vi "Quadrotor RT.vi"() -> ()   [LabVIEW 2015]
uses:
  <vilib>/Platform/TimedLoop/XDataNode/timing_clust.ctl
  <vilib>/Platform/TimedLoop/XDataNode/nitl_modes.ctl
  <vilib>/Platform/TimedLoop/XDataNode/wakeup.ctl
  <vilib>/FPGAPlugInAG/myRIO-1900/niLvFpga_Open_myRIO-1900.vi
  <vilib>/rvi/interface/common/dynamic/niFpgaDynamicAddResources.vi
  <vilib>/myRIO/Common/Instrument Driver Framework/Utilities/vis/FPGA Ref Manager.vi
  <vilib>/Utility/error.llb/Error Cluster From Error Code.vi
  <vilib>/myRIO/Common/Instrument Driver Framework/Utilities/vis/Ref Counter.vi
  <vilib>/Utility/xml.llb/Read From XML File(string).vi
  <vilib>/Utility/xml.llb/Write to XML File(string).vi
  <vilib>/FPGAPlugInAG/Dynamic/niLvFpga_Close_Dynamic.vi
  <vilib>/rvi/interface/nirviOpenFPGA/nirviOpenFPGA.xnode
  FPGA Bitfiles/MyThirdNImyRIOPr_FPGATarget_myRIO-1900Quadro_oM0Jv1TSYjE.lvbitx
  <vilib>/Platform/TimedLoop/XDataNode/XDataNode.xnode
  <vilib>/rvi/interface/nirviCloseFPGA/nirviCloseFPGA.xnode
  <vilib>/Platform/TimedLoop/XDataNode/XDNodeRunTimeDep.lvlib
  <vilib>/myRIO/Instrument Drivers/Utilities/Utilities.lvlib
panel:
  out "Buffer In":u8[](array[numeric])=[204, 0, 0, 0, 0, 0, 0, 0, 0, 0, 0, 0, 0, 0, 0, 0, 0, 0, 0, 0, 0, 0, 0, 0, 0, 0, 0, 0, 0, 0, 0, 0, 85, 170] format="0x%x"
  in  "停止调试":bool
  out "roll":dbl(knob) scale=-90.0..90.0
  out "陀螺仪积分时间间隔":sgl(graph)=0.002
  in  "D":dbl(slide)=45.4945 scale=0.0..300.0
  in  "P":dbl(slide)=50.5495 scale=0.0..500.0
  in  "I":dbl(slide)=0.013 scale=0.0..5.0
  in  "Yaw_D":dbl=10.0
  in  "Yaw_I":dbl
  in  "Yaw_P":dbl=200.0
  in  "滑动杆":dbl(slide)=-0.061919504643962814 scale=-10.0..10.0
  out "Pitch: 控制\\反馈":cluster{sgl, "Pitch":dbl}(graph)
  out "Roll: 控制\\反馈":cluster{sgl, "Roll":dbl}(graph)
  out "Yaw: 控制\\反馈":cluster{"GYR_I_Z":sgl}(graph)
  out "Roll计算后数值":dbl
  out "Pitch计算后数值":dbl
  out "Yaw计算后数值":dbl
  out "输出簇":T1(graph)
  in  "ACCADJ":T2
  out "GYR_I_X":sgl
  out "GYR_I_Y":sgl
  out "AccMean":T2={"ACC_OFFSET_X"=63.977, "ACC_OFFSET_Y"=220.058, "ACC_OFFSET_Z"=0.0}
  out "GyrMean":T3
  out "摇杆按键 9":bool[](array[boolean])
  out "摇杆按键 8":bool[](array[boolean])
  out "摇杆按键 7":bool[](array[boolean])
  out "摇杆按键 6":bool[](array[boolean])
  out "摇杆按键 5":bool[](array[boolean])
  out "摇杆按键 4":bool[](array[boolean])
  out "摇杆按键 3":bool[](array[boolean])
  out "摇杆按键 2":bool[](array[boolean])
  out "油门":u16(knob) scale=0.0..20000.0
  out "X axis":i32(slide) scale=-32768.0..32767.0
  out "Y axis":i32(slide) scale=-32768.0..32767.0
  out "小方向":u8
  out "摇杆按键":bool[](array[boolean])
  out "XY图":cluster{i32[], i32[]}(graph)
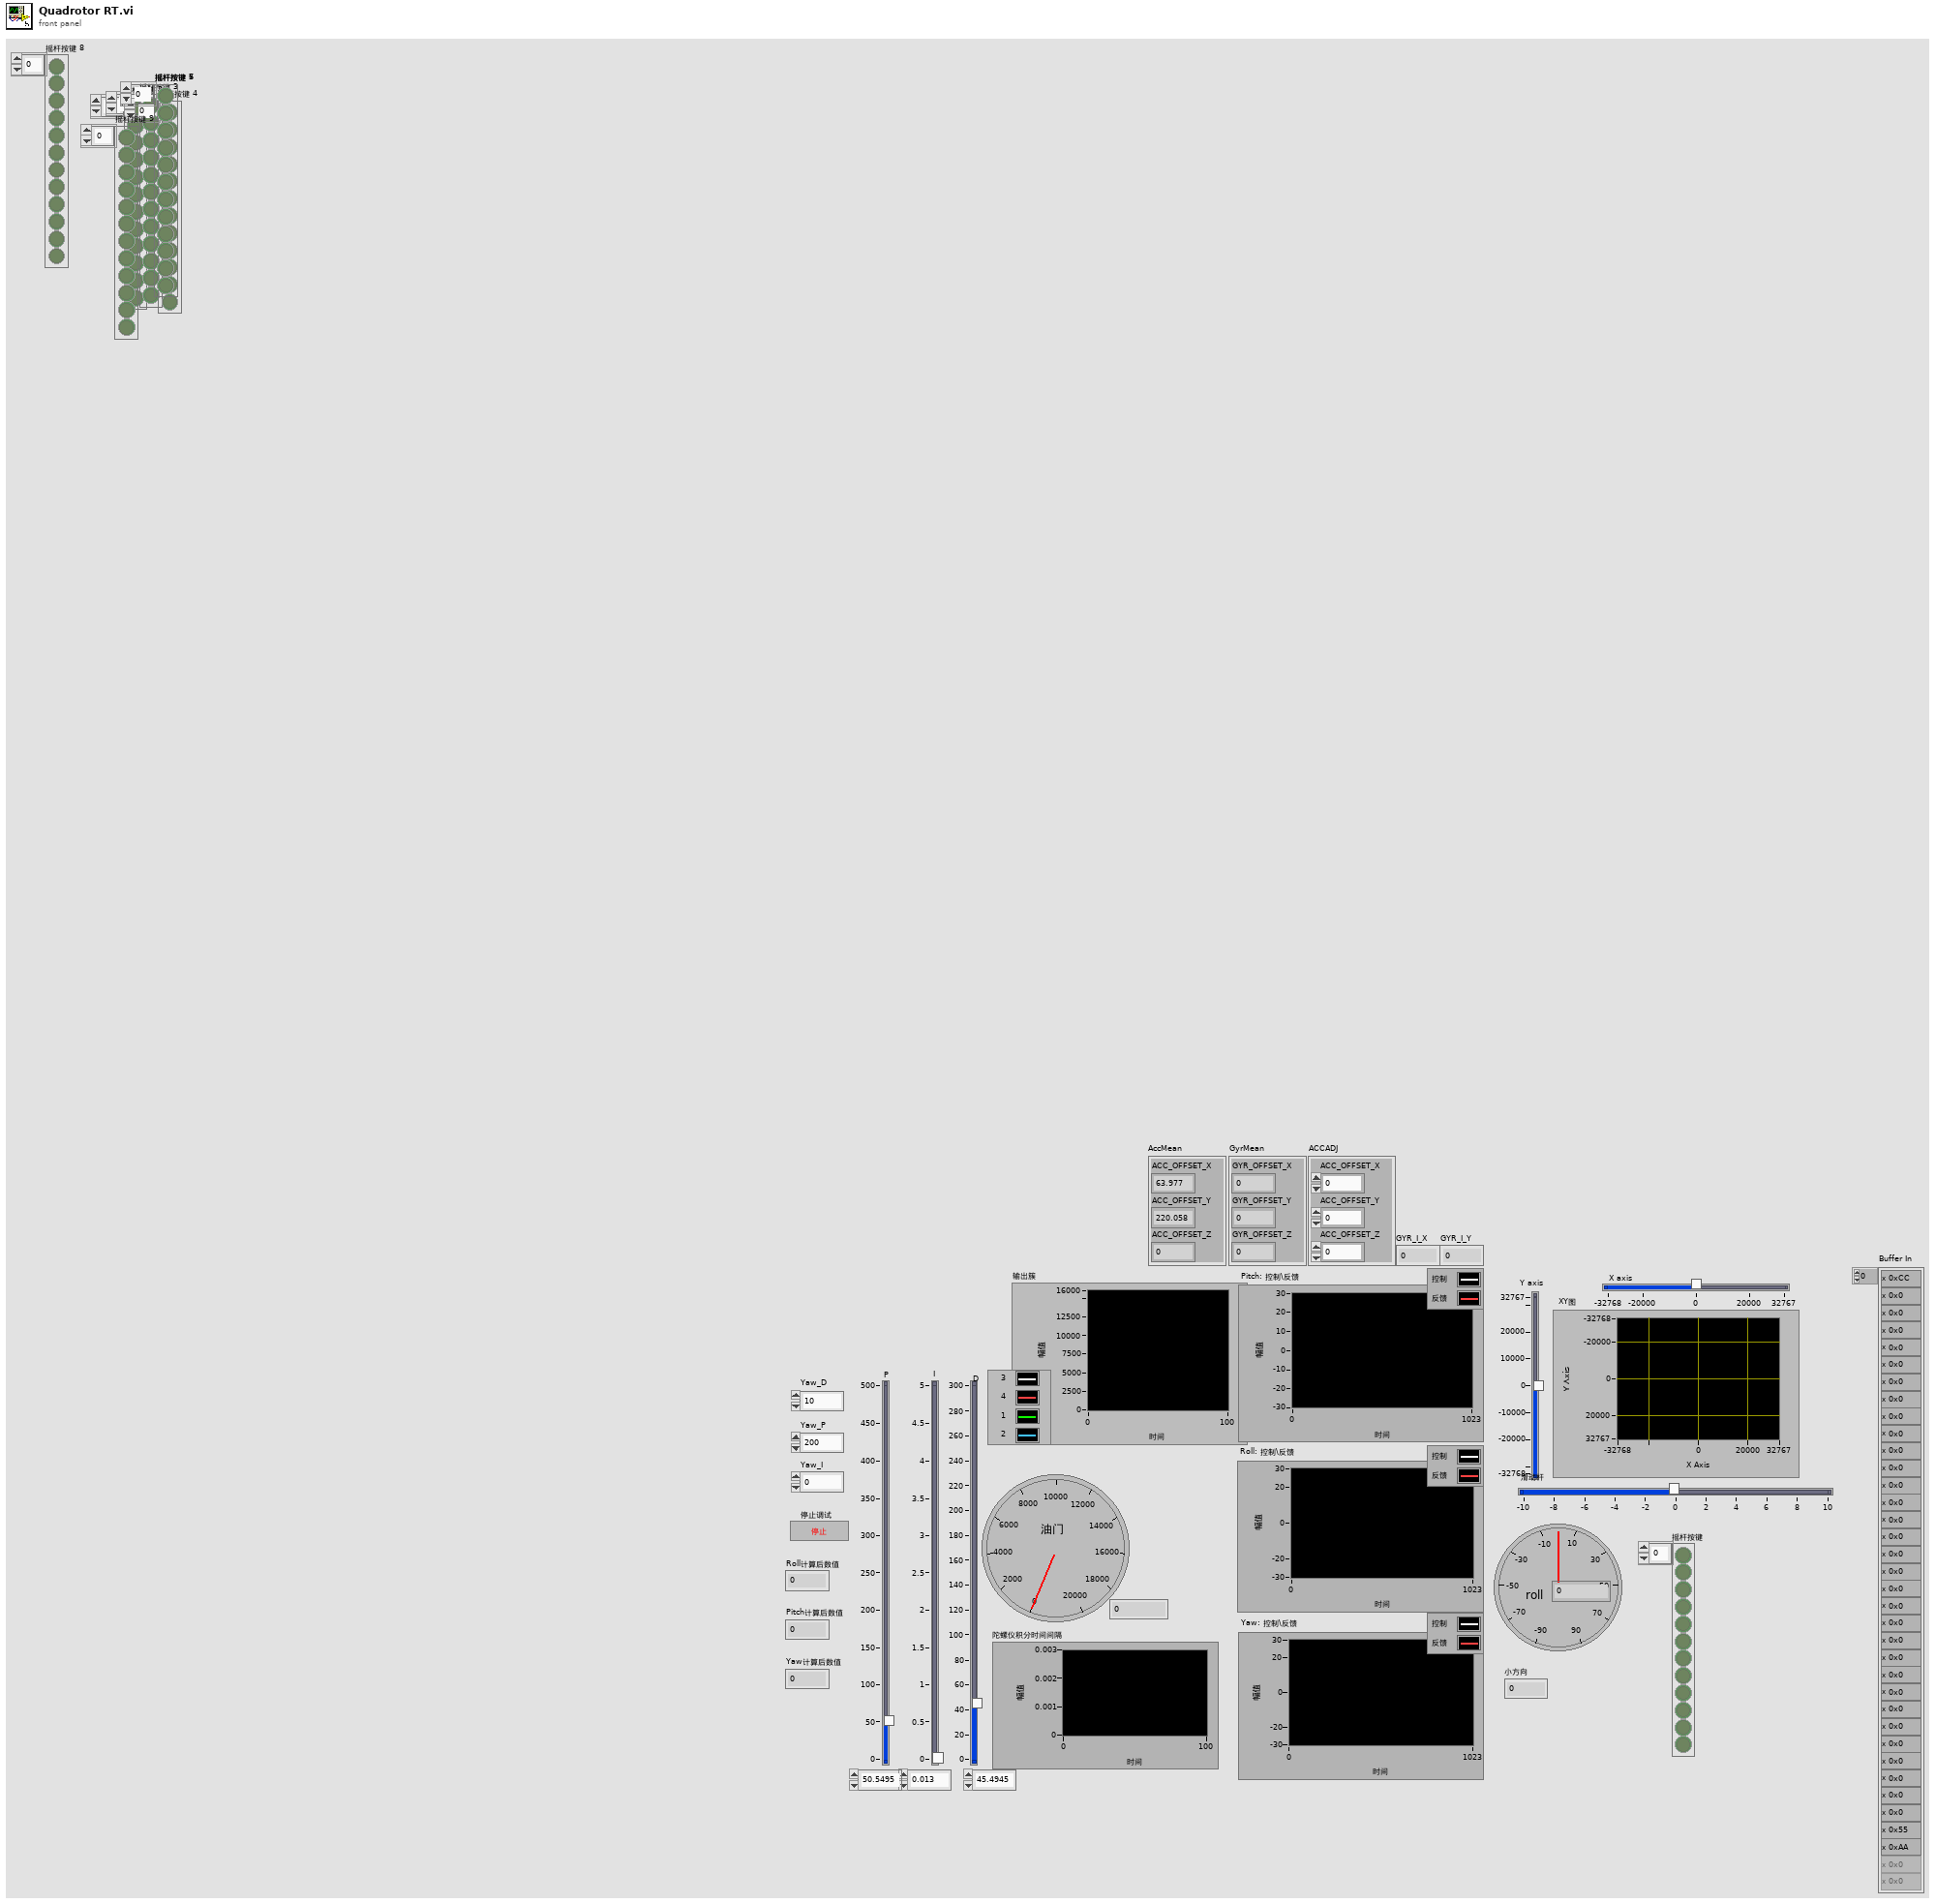
[diagram p1: front panel]
types:
  T1 = cluster{"PWM0":u16, "PWM1":u16, "PWM2":u16, "PWM3":u16}
  T2 = cluster{"ACC_OFFSET_X":sgl, "ACC_OFFSET_Y":sgl, "ACC_OFFSET_Z":sgl}
  T3 = cluster{"GYR_OFFSET_X":sgl, "GYR_OFFSET_Y":sgl, "GYR_OFFSET_Z":sgl}
  T4 = cluster{"输入簇":cluster{"ACC_OFFSET_X":sgl, "ACC_OFFSET_Y":sgl, "ACC_OFFSET_Z":sgl}, "输入簇":cluster{"GYR_OFFSET_X":sgl, "GYR_OFFSET_Y":sgl, "GYR_OFFSET_Z":sgl}}
  T5 = typedef "XDNodeRunTimeDep.lvlib/timing_clust.ctl" = cluster{"Expected End [f-1]":u64, "Actual End [f-1]":u64, "Finished Late? [f-1]":bool, "Expected End [i-1]":u64, "Actual End [i-1]":u64, "Finished Late? [i-1]":bool, "Expected Start [i]":u64, "Actual Start [i]":u64, "Expected Start [f]":u64, "Actual Start [f]":u64, "Source Name":string, "Structure Name":string, "Period":i64, "Deadline":i64, "Offset":i64, "Start":i64, "Priority":i32, "Timeout":i32, "Mode":T6, "Wakeup Reason":T7, "Error":errorcluster, "Source Type":string, "Secondary Source Type":string, "Global End Time":u64, "Global Start Time":u64, "Frame Duration":u64, "Iteration Duration":u64, "Assigned CPU":i32, "I/O Scan Engine Mode":u32}
  T6 = typedef "XDNodeRunTimeDep.lvlib/nitl_modes.ctl" = enum32{"No Change", "Process missed periods, maintain original phase", "Discard missed periods, maintain original phase", "Process missed periods, ignore original phase", "Discard missed periods, ignore original phase"}
  T7 = typedef "XDNodeRunTimeDep.lvlib/wakeup.ctl" = enum32{"Normal", "Aborted", "Asynchronous wakeup", "Timing source error", "Timed loop error", "Timeout"}
  T8 = cluster{"EI_Roll":sgl, "EI_Pitch":sgl, "EI_Yaw":sgl}
  T9 = cluster{"q0":dbl, "q1":dbl, "q2":dbl, "q3":dbl, "exInt":dbl, "eyInt":dbl, "ezInt":dbl}
  T10 = cluster{"GYR_I_X":sgl, "GYR_I_Y":sgl, "GYR_I_Z":sgl, "t":sgl}
  T11 = cluster{"DataX":sgl[], "DataY":sgl[], "DataZ":sgl[], "Num":i32, "Cnt":i32}
  T12 = cluster{"ACC_AVG_X":sgl, "ACC_AVG_Y":sgl, "ACC_AVG_Z":sgl}
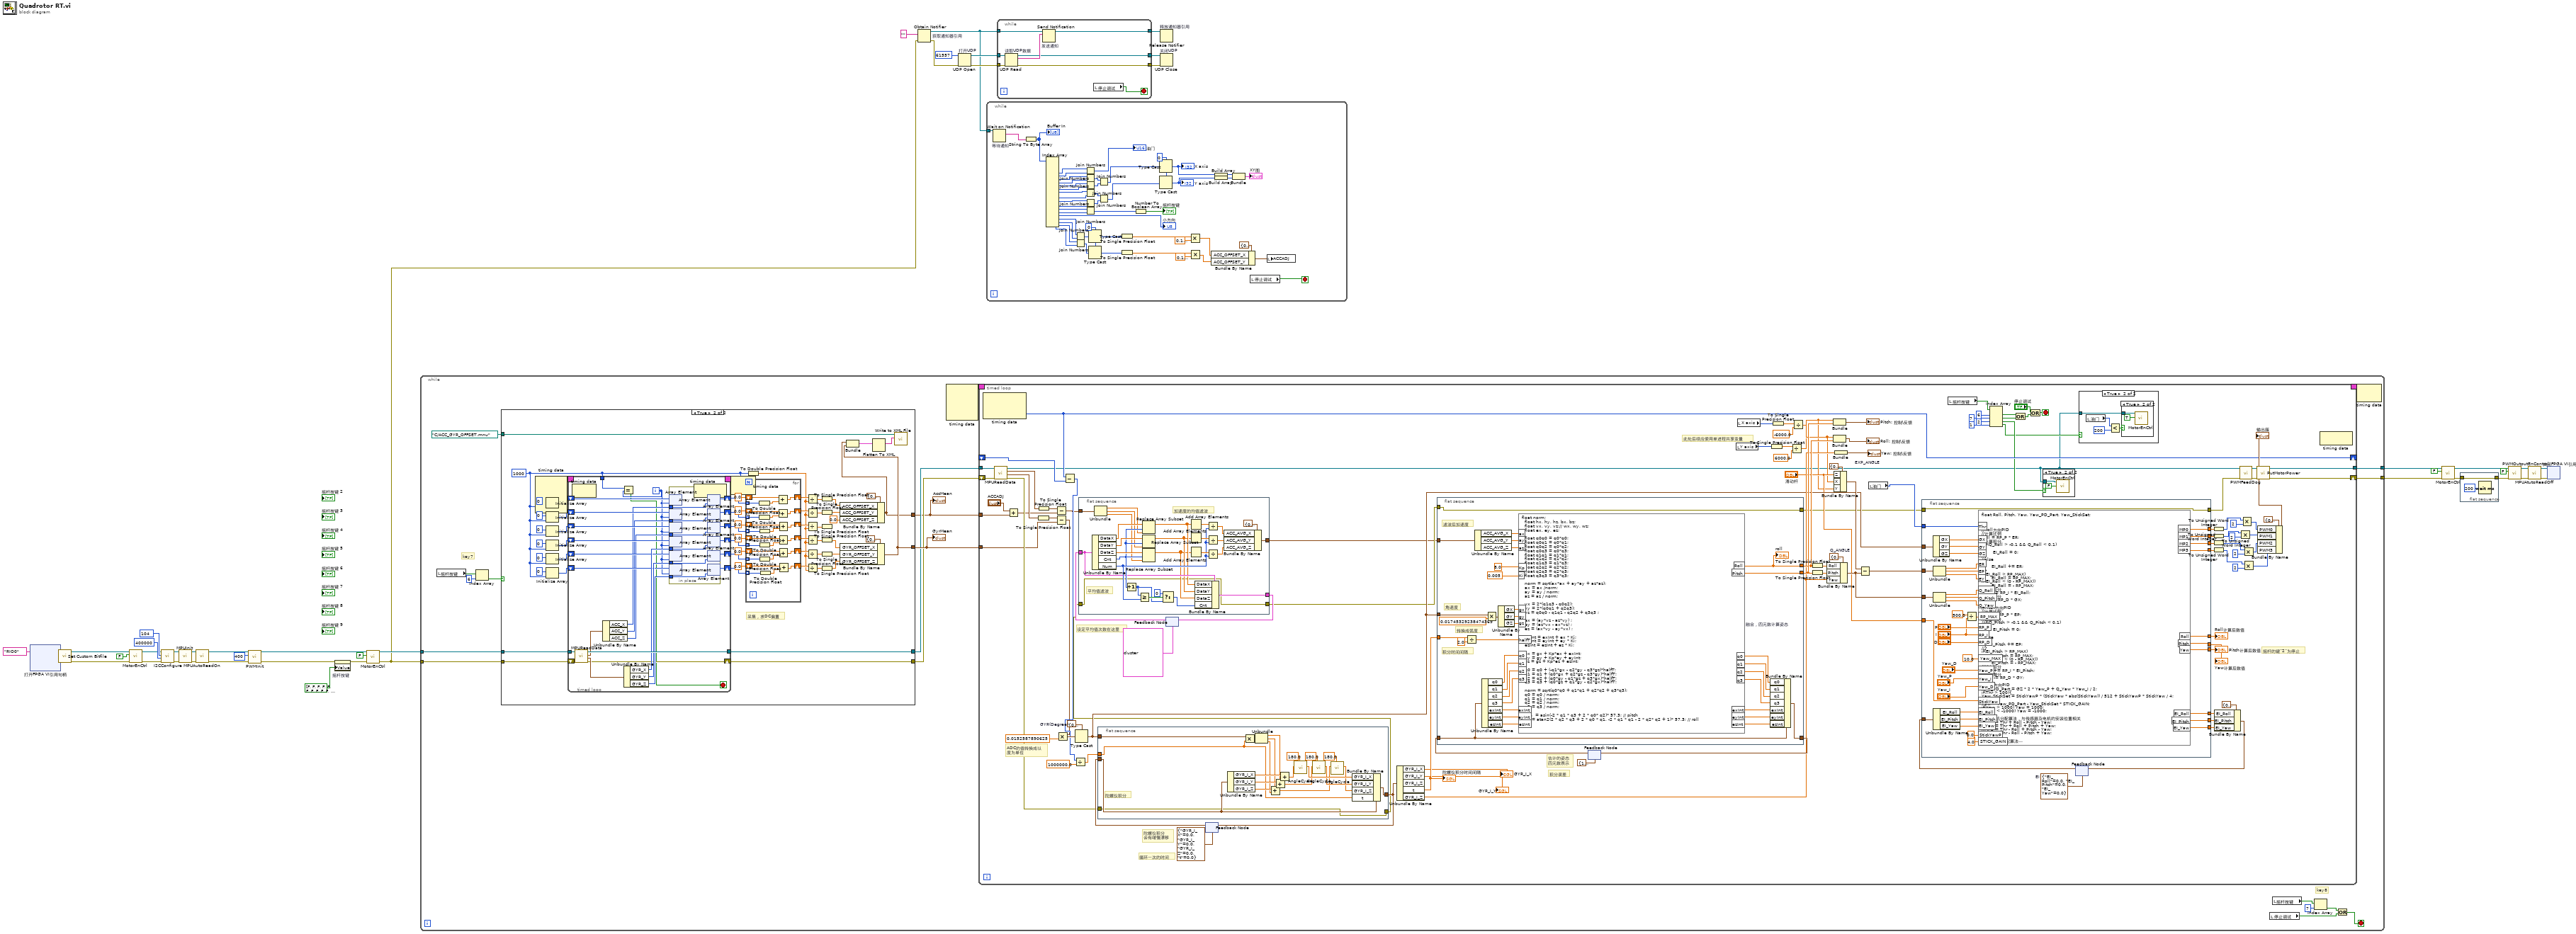
[diagram p0: block diagram]
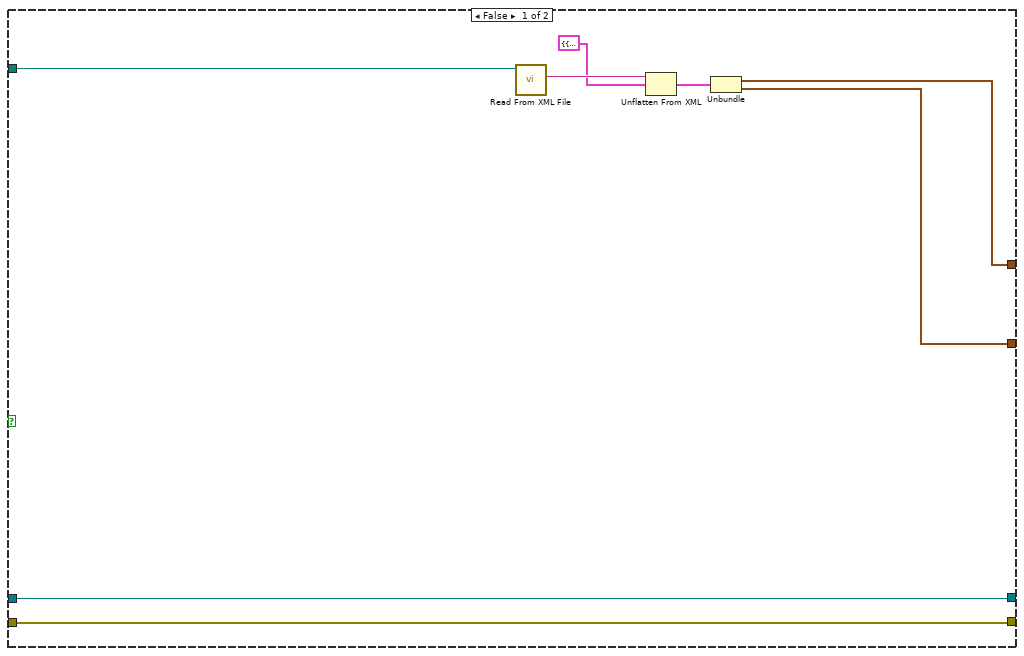
[diagram p2: hidden frame]
diagram:
  n1 = xnode "打开FPGA VI引用句柄"("资源名称"=tag "RIO0" ("resource name")) -> ("FPGA VI引用输出"=w3:refnum<k20>, "错误输出"=w4:errorcluster)  [unwired: 1 in]
  n2 = call <vilib>:"Set Custom Bitfile.vi"("error in (no error)"=w4, "Custom FPGA Reference In"=w3) -> ("error out"=w2:errorcluster, "Custom FPGA Reference Out"=w1:refnum<k20>)  [unwired: 8 in]
  n3 = call "MotorEnCtrl.vi"("ErrorIn(no error)"=w2, "MotorEN?(F)"=FALSE, "FPGA VI引用输入"=w1) -> ("ErrorOut"=w31:errorcluster, "FPGA VI引用输出"=w32:refnum<k20>)  [unwired: 7 in]
  n4 = call "I2CConfigure.vi"("error in (no error)"=w31, "Clock Rate"=u32 400000, "IICSlaveAddress"=u16 104, "FPGA VI引用输入"=w32) -> ("error out"=w43:errorcluster, "FPGA VI引用输出"=w44:refnum<k20>)  [unwired: 6 in]
  n5 = call "MPUInit.vi"("ErrorIn(no error)"=w43, "FPGA VI引用输入"=w44) -> ("ErrorOut"=w41:errorcluster, "FPGA VI引用输出"=w42:refnum<k20>)  [unwired: 8 in]
  n6 = call "MPUAutoReadOn.vi"("ErrorIn(no error)"=w41, "FPGA VI引用输入"=w42) -> ("ErrorOut"=w19:errorcluster, "FPGA VI引用输出"=w18:refnum<k20>)  [unwired: 8 in]
  n7 = call "PWMInit.vi"("ErrorIn(no error)"=w19, "PMWFreq(200Hz)"=u32 400, "FPGA VI引用输入"=w18) -> ("ErrorOut"=w16:errorcluster, "FPGA VI引用输出"=w17:refnum<k20>)  [unwired: 7 in]
  n8 = property on="摇杆按键" class="Arr (strict)"(error in=w16, "Value"=bool[] [FALSE, FALSE, FALSE, FALSE, FALSE, FALSE, FALSE, FALSE, FALSE, FALSE, FALSE, FALSE, FALSE, FALSE, FALSE, FALSE] ("输出数组")) -> (error out=w22:errorcluster)  [unwired: 1 in, 1 out]
  n9 = call "MotorEnCtrl.vi"("ErrorIn(no error)"=w22, "MotorEN?(F)"=FALSE, "FPGA VI引用输入"=w17) -> ("ErrorOut"=w6:errorcluster, "FPGA VI引用输出"=w20:refnum<k20>)  [unwired: 7 in]
  n10 = while {
    tunnel: [w61] -> w29
    tunnel: [w60] -> w28
    tunnel: w20 -> [w56]
    tunnel: w6 -> [w55]
    stop <- w47 stop-if-true
    # "key7"
    # "key8"
    n11 = local read "摇杆按键"() -> (w53:bool[])
    n12 = Index Array(array=w53, index=6 ("索引")) -> (element=w51:bool)
    n13 = case shown="True" w51 {
      tunnel: [w65 w74] -> w59
      tunnel: [w71 w80] -> w58
      tunnel: [w70 w79] -> w57
      tunnel: w56 -> [w71 w78]
      tunnel: w55 -> [w70 w77]
      tunnel: path "C:/ACC_GYR_OFFSET.mnu" ("XML File Path") -> [w69 w76]
      tunnel: [w64 w72] -> w45
      frame False {
        n14 = call-poly <vilib>:"Read From XML File.vi"("XML File Path"=w69) -> ("XML Elements"=w68:string)  [unwired: 8 in, 2 out]
        n15 = Unflatten From XML(xml string=w68, type=T4 {"输入簇"={"ACC_OFFSET_X"=0.0, "ACC_OFFSET_Y"=0.0, "ACC_OFFSET_Z"=0.0}, "输入簇"={"GYR_OFFSET_X"=0.0, "GYR_OFFSET_Y"=0.0, "GYR_OFFSET_Z"=0.0}} ("输出簇")) -> (value=w66:T4)  [unwired: 1 in, 1 out]
        n16 = Unbundle(w66) -> ("输入簇"=w64:T2, "输入簇"=w65:T3)
      }
      frame True {
        w81 = 1000
        # "采集，求DC偏置"
        n17 = node-c288() -> (w128:T5)  [unwired: 4 in]
        n18 = Initialize Array(i16 0 ("元素"), w81) -> (w102:i16[])
        n19 = Initialize Array(i16 0 ("元素"), w81) -> (w120:i16[])
        n20 = Initialize Array(i16 0 ("元素"), w81) -> (w119:i16[])
        n21 = Initialize Array(i16 0 ("元素"), w81) -> (w118:i16[])
        n22 = Initialize Array(i16 0 ("元素"), w81) -> (w117:i16[])
        n23 = Initialize Array(i16 0 ("元素"), w81) -> (w116:i16[])
        n24 = timed-loop {
          tunnel: [w154] -> w80
          shift-right: [w143] -> w101
          shift-left: w102 -> [w152]
          shift-right: [w142] -> w100
          shift-left: w120 -> [w151]
          shift-right: [w141] -> w99
          shift-left: w119 -> [w150]
          shift-right: [w140] -> w98
          shift-left: w118 -> [w149]
          shift-right: [w139] -> w97
          shift-left: w117 -> [w147]
          shift-right: [w138] -> w96
          shift-left: w116 -> [w145]
          shift-right: [w133] -> w79
          shift-left: w77 -> [w155]
          timing: w128 -> [_]
          timing-out: [_] -> w127
          tunnel: w81 -> [w132]
          tunnel: w78 -> [w129]
          i -> [w131]
          stop <- w130 stop-if-true
          n25 = node-c288() -> ()  [unwired: 1 in, 1 out]
          n26 = call "MPUReadData.vi"("ErrorIn"=w155, "FPGA VI引用输入"=w129) -> ("ErrorOut"=w133:errorcluster, "GYR"=w153:cluster{"GYR_X":i16, "GYR_Y":i16, "GYR_Z":i16}, "ACC"=w137:cluster{"ACC_X":i16, "ACC_Y":i16, "ACC_Z":i16}, "FPGA VI引用输出"=w154:refnum<k20>)  [unwired: 5 in, 1 out]
          n27 = Unbundle By Name(w137) -> ("ACC_X"=w136:i16, "ACC_Y"=w135:i16, "ACC_Z"=w134:i16)
          n28 = Equal?(x=w132, y=w131) -> (x = y?=w130:bool)
          n29 = Unbundle By Name(w153) -> ("GYR_X"=w148:i16, "GYR_Y"=w146:i16, "GYR_Z"=w144:i16)
          n30 = in-place {
            in-place-border: w136 -> [w163]
            in-place-border: w135 -> [w162]
            in-place-border: w134 -> [w161]
            in-place-border: w148 -> [w160]
            in-place-border: w146 -> [w159]
            in-place-border: w144 -> [w158]
            n31 = in-place-array #1(w152, w131) -> ()  [unwired: 1 out]
            n32 = in-place-array #2(w151, w131) -> ()  [unwired: 1 out]
            n33 = in-place-array #3(w150, w131) -> ()  [unwired: 1 out]
            n34 = in-place-array #4(w149, w131) -> ()  [unwired: 1 out]
            n35 = in-place-array #5(w147, w131) -> ()  [unwired: 1 out]
            n36 = in-place-array #6(w145, w131) -> ()  [unwired: 1 out]
            n37 = in-place-array #1(w163) -> (w143:i16[])  [unwired: 1 out]
            n38 = in-place-array #2(w162) -> (w142:i16[])  [unwired: 1 out]
            n39 = in-place-array #3(w161) -> (w141:i16[])  [unwired: 1 out]
            n40 = in-place-array #4(w160) -> (w140:i16[])  [unwired: 1 out]
            n41 = in-place-array #5(w159) -> (w139:i16[])  [unwired: 1 out]
            n42 = in-place-array #6(w158) -> (w138:i16[])  [unwired: 1 out]
          }
          n43 = node-c288() -> ()  [unwired: 1 in, 1 out]
        }
        n44 = node-c288(w127) -> ()  [unwired: 1 out]
        n45 = for {
          N: w81 -> [_]
          tunnel: w101 -> [w189] mode=indexing
          tunnel: w100 -> [w180] mode=indexing
          tunnel: w99 -> [w177] mode=indexing
          tunnel: w98 -> [w174] mode=indexing
          tunnel: w97 -> [w172] mode=indexing
          tunnel: w96 -> [w170] mode=indexing
          shift-right: [w186] -> w109
          shift-left: 0.0 -> [w188]
          shift-right: [w178] -> w108
          shift-left: 0.0 -> [w179]
          shift-right: [w175] -> w107
          shift-left: 0.0 -> [w176]
          shift-right: [w166] -> w106
          shift-left: 0.0 -> [w173]
          shift-right: [w167] -> w105
          shift-left: 0.0 -> [w171]
          shift-right: [w168] -> w104
          shift-left: 0.0 -> [w169]
          n46 = To Double Precision Float(number=w189) -> (double precision float=w187:dbl)
          n47 = To Double Precision Float(number=w180) -> (double precision float=w185:dbl)
          n48 = To Double Precision Float(number=w177) -> (double precision float=w184:dbl)
          n49 = To Double Precision Float(number=w174) -> (double precision float=w183:dbl)
          n50 = To Double Precision Float(number=w172) -> (double precision float=w182:dbl)
          n51 = To Double Precision Float(number=w170) -> (double precision float=w181:dbl)
          n52 = Add(x=w188, y=w187) -> (x+y=w186:dbl)
          n53 = Add(x=w179, y=w185) -> (x+y=w178:dbl)
          n54 = Add(x=w176, y=w184) -> (x+y=w175:dbl)
          n55 = Add(x=w173, y=w183) -> (x+y=w166:dbl)
          n56 = Add(x=w171, y=w182) -> (x+y=w167:dbl)
          n57 = Add(x=w169, y=w181) -> (x+y=w168:dbl)
        }
        n58 = To Double Precision Float(number=w81) -> (double precision float=w103:dbl)
        n59 = Divide(x=w109, y=w103) -> (x/y=w94:dbl)
        n60 = Divide(x=w108, y=w103) -> (x/y=w93:dbl)
        n61 = Divide(x=w107, y=w103) -> (x/y=w92:dbl)
        n62 = Divide(x=w106, y=w103) -> (x/y=w91:dbl)
        n63 = Divide(x=w105, y=w103) -> (x/y=w90:dbl)
        n64 = Divide(x=w104, y=w103) -> (x/y=w89:dbl)
        n65 = To Single Precision Float(number=w94) -> (single precision float=w88:sgl)
        n66 = To Single Precision Float(number=w93) -> (single precision float=w87:sgl)
        n67 = To Single Precision Float(number=w92) -> ()  [unwired: 1 out]
        n68 = To Single Precision Float(number=w91) -> (single precision float=w85:sgl)
        n69 = To Single Precision Float(number=w90) -> (single precision float=w84:sgl)
        n70 = To Single Precision Float(number=w89) -> (single precision float=w83:sgl)
        n71 = Bundle By Name(cluster=T2 {"ACC_OFFSET_X"=0.0, "ACC_OFFSET_Y"=0.0, "ACC_OFFSET_Z"=0.0} ("输入簇"), "ACC_OFFSET_X"=w88, "ACC_OFFSET_Y"=w87, "ACC_OFFSET_Z"=sgl 0.0) -> (w72:T2)
        n72 = Bundle By Name(cluster=T3 {"GYR_OFFSET_X"=0.0, "GYR_OFFSET_Y"=0.0, "GYR_OFFSET_Z"=0.0} ("输入簇"), "GYR_OFFSET_X"=w85, "GYR_OFFSET_Y"=w84, "GYR_OFFSET_Z"=w83) -> (w74:T3)
        n73 = Bundle("输入簇"=w72, "输入簇"=w74) -> (w73:T4)  [unwired: 1 in]
        n74 = Flatten To XML(anything=w73) -> (xml string=w75:string)
        n75 = call-poly <vilib>:"Write to XML File.vi"("XML Input"=w75, "XML File Path"=w76) -> ()  [unwired: 7 in, 3 out]
      }
    }
    "AccMean" <- w45
    "GyrMean" <- w59
    n76 = node-c288() -> (w63:T5)  [unwired: 4 in]
    n77 = timed-loop {
      timing: w63 -> [_]
      timing-out: [_] -> w62
      tunnel: w58 -> [w296]
      tunnel: w45 -> [w227]
      tunnel: w59 -> [w224]
      tunnel: [w209] -> w61
      shift-right: [w277] -> w60
      shift-left: w57 -> [w283]
      shift-right: [w208] -> _
      shift-left: _ -> [w242]
      stop <- w234 stop-if-true
      w260 = cluster{"X":sgl, "Y":sgl, "Z":sgl} {"X"=0.0, "Y"=0.0, "Z"=0.0}  # EXP_ANGLE
      w272 = T8 {"EI_Roll"=0.0, "EI_Pitch"=0.0, "EI_Yaw"=0.0}  # EI
      w280 = cluster{"GX":sgl, "GY":sgl, "GZ":sgl} {"GX"=0.0, "GY"=0.0, "GZ"=0.0}  # GYR(Degree)
      w281 = cluster{"Roll":sgl, "Pitch":sgl, "Yaw":sgl} {"Roll"=0.0, "Pitch"=0.0, "Yaw"=0.0}  # Q_ANGLE
      # "此处后续应使用单进程共享变量"
      # "摇杆的键“2”为停止"
      # "循环一次的时间"
      # "陀螺仪积分\n会有缓慢漂移"
      # "估计的姿态\n四元数表示"
      # "积分误差"
      # "ADC的值转换成以\n度为单位"
      # "设定平均值次数在这里"
      n78 = node-c288() -> (w208:i64)  [unwired: 1 in, 2 out]
      n79 = call "MPUReadData.vi"("ErrorIn"=w283, "FPGA VI引用输入"=w296) -> ("ErrorOut"=w246:errorcluster, "GYR"=w250:cluster{"GYR_X":i16, "GYR_Y":i16, "GYR_Z":i16}, "ACC"=w231:cluster{"ACC_X":i16, "ACC_Y":i16, "ACC_Z":i16}, "FPGA VI引用输出"=w205:refnum<k20>)  [unwired: 5 in, 1 out]
      n80 = Add(x="ACCADJ", y=w227) -> (x+y=w226:T2)
      n81 = To Single Precision Float(number=w250) -> (single precision float=w294:cluster{"GYR_X":sgl, "GYR_Y":sgl, "GYR_Z":sgl})
      n82 = To Single Precision Float(number=w231) -> (single precision float=w295:cluster{"ACC_X":sgl, "ACC_Y":sgl, "ACC_Z":sgl})
      n83 = Subtract(x=w295, y=w226) -> (x-y=w228:cluster{sgl, sgl, sgl})
      n84 = Subtract(x=w294, y=w224) -> (x-y=w229:cluster{sgl, sgl, sgl})
      n85 = Multiply(x=w229, y=sgl 0.015258789) -> (x*y=w248:cluster{sgl, sgl, sgl})
      n86 = Subtract(x=w208, y=w242) -> (x-y=w241:i64)
      n87 = Divide(x=w241, y=sgl 1000000.0) -> (x/y=w239:sgl)
      n88 = Type Cast(type=w280, x=w248) -> (*(type *) &x=w247:cluster{"GX":sgl, "GY":sgl, "GZ":sgl})
      n89 = flat-sequence {
        tunnel: w292 -> [w406]
        tunnel: w228 -> [w415]
        tunnel: [w407] -> w230
        tunnel: [w401] -> w291
        tunnel: w245 -> [w400]
        tunnel: [w400] -> w244
        frame #0 {
          # "加速度的均值滤波"
          # "平均值滤波"
          n90 = Unbundle By Name(w406) -> ("DataX"=w419:sgl[], "DataY"=w418:sgl[], "DataZ"=w426:sgl[], "Cnt"=w416:i32, "Num"=w417:i32)
          n91 = Unbundle(w415) -> (w412:sgl, w413:sgl, w414:sgl)
          n92 = Increment(x=w416) -> (x+1=w422:i32)
          n93 = Greater Or Equal?(x=w422, y=w417) -> (x >= y?=w424:bool)
          n94 = Replace Array Subset(array=w419, new element=w412, index=w416) -> (w405:sgl[])
          n95 = Replace Array Subset(array=w418, new element=w413, index=w416) -> (w404:sgl[])
          n96 = Replace Array Subset(array=w426, new element=w414, index=w416) -> (w403:sgl[])
          n97 = Select(t=0, s=w424, f=w422) -> (s? t:f=w402:i32)
          n98 = Add Array Elements ("数组元素相加")(numeric array=w405) -> (sum=w421:sgl)
          n99 = Add Array Elements(numeric array=w404) -> (sum=w420:sgl)
          n100 = Add Array Elements(numeric array=w403) -> (sum=w425:sgl)
          n101 = Bundle By Name(cluster=w406, "DataX"=w405, "DataY"=w404, "DataZ"=w403, "Cnt"=w402) -> (w401:T11)
          n102 = Divide(x=w421, y=w417) -> (x/y=w410:sgl)
          n103 = Divide(x=w420, y=w417) -> (x/y=w409:sgl)
          n104 = Divide(x=w425, y=w417) -> (x/y=w408:sgl)
          n105 = Bundle By Name(cluster=T12 {"ACC_AVG_X"=0.0, "ACC_AVG_Y"=0.0, "ACC_AVG_Z"=0.0} ("输入簇"), "ACC_AVG_X"=w410, "ACC_AVG_Y"=w409, "ACC_AVG_Z"=w408) -> (w407:T12)
        }
      }
      n106 = flat-sequence {
        tunnel: w288 -> [w390]
        tunnel: w247 -> [w399]
        tunnel: [w391] -> w284
        tunnel: [w380] -> w245
        tunnel: w246 -> [w380]
        tunnel: w239 -> [w379]
        frame #0 {
          # "陀螺仪积分"
          n107 = Unbundle By Name(w390) -> ("GYR_I_X"=w397:sgl, "GYR_I_Y"=w395:sgl, "GYR_I_Z"=w393:sgl)
          n108 = Multiply(x=w399, y=w379) -> (x*y=w398:cluster{"GX":sgl, "GY":sgl, "GZ":sgl})
          n109 = Unbundle(w398) -> ("GX"=w396:sgl, "GY"=w394:sgl, "GZ"=w392:sgl)
          n110 = Add(x=w393, y=w392) -> (x+y=w383:sgl)
          n111 = Add(x=w395, y=w394) -> (x+y=w385:sgl)
          n112 = Add(x=w397, y=w396) -> (x+y=w389:sgl)
          n113 = call "AngleCycle.vi"("MAX"=sgl 180.0, "Angle"=w389) -> ("AngleOut"=w387:sgl)  [unwired: 9 in]
          n114 = call "AngleCycle.vi"("MAX"=sgl 180.0, "Angle"=w385) -> ("AngleOut"=w384:sgl)  [unwired: 9 in]
          n115 = call "AngleCycle.vi"("MAX"=sgl 180.0, "Angle"=w383) -> ("AngleOut"=w382:sgl)  [unwired: 9 in]
          n116 = Bundle By Name(cluster=w390, "GYR_I_X"=w387, "GYR_I_Y"=w384, "GYR_I_Z"=w382, "t"=w379) -> (w391:T10)
        }
      }
      n117 = feedback-in #7(w291) -> ()
      n118 = feedback #7(T11 {"DataX"=array[1001 elements], "DataY"=array[1001 elements], "DataZ"=array[1001 elements], "Num"=30, "Cnt"=0}) -> (w292:T11)
      n119 = feedback-in #8(w284) -> ()
      n120 = feedback #8(T10 {"GYR_I_X"=0.0, "GYR_I_Y"=0.0, "GYR_I_Z"=0.0, "t"=0.0}) -> (w288:T10)
      n121 = Unbundle By Name(w284) -> ("GYR_I_X"=→"GYR_I_X":sgl, "GYR_I_Y"=→"GYR_I_Y":sgl, "t"=w282:sgl, "GYR_I_Z"=w249:sgl)  [unwired: 1 out]
      "陀螺仪积分时间间隔" <- w282
      n122 = flat-sequence {
        tunnel: [w371] -> w285
        tunnel: [w347] -> w254
        tunnel: [w352] -> w257
        tunnel: w286 -> [w372]
        tunnel: w230 -> [w349]
        tunnel: w247 -> [w359]
        tunnel: w282 -> [w355]
        tunnel: w244 -> [w348]
        tunnel: [w348] -> w202
        frame #0 {
          # "积分时间间隔"
          # "角速度"
          # "滤波后加速度"
          # "转换成弧度"
          n123 = Divide(x=w355, y=sgl 2.0) -> (x/y=w354:sgl)
          n124 = Unbundle By Name(w349) -> ("ACC_AVG_X"=w351:sgl, "ACC_AVG_Y"=w356:sgl, "ACC_AVG_Z"=w362:sgl)
          n125 = Unbundle By Name(w372) -> ("q0"=w363:dbl, "q1"=w378:dbl, "q2"=w377:dbl, "q3"=w376:dbl, "exInt"=w375:dbl, "eyInt"=w374:dbl, "ezInt"=w373:dbl)
          n126 = Multiply(x=w359, y=sgl 0.017453292) -> (x*y=w358:cluster{"GX":sgl, "GY":sgl, "GZ":sgl})
          n127 = Unbundle By Name(w358) -> ("GX"=w350:sgl, "GY"=w361:sgl, "GZ"=w360:sgl)
          n128 = formula code="float norm;\n  float hx, hy, hz, bx, bz;\n  float vx, vy, vz;// wx, wy, wz;\n  float ex, ey, ez;\n\n  float q0q0 = q0*q0;\n  float q0q1 = q0*q1;\n  float q0q2 = q0*q2;\n  float q0q3 = q0*q3;\n  float q1q1 = q1*q1;\n  float q1q2 = q1*q2;\n  float q1q3 = q1*q3;\n  float q2q2 = q2*q2;\n  float q2q3 = q2*q3;\n  float q3q3 = q3*q3;\n\n  norm = sqrt(ax*ax + ay*ay + az*az);      \n  ax = ax /norm;\n  ay = ay / norm;\n  az = az / norm;\n           \n  vx = 2*(q1q3 - q0q2);\t\t\t\t\t\t\t\t\t\t\t\t\n  vy = 2*(q0q1 + q2q3);\n  vz = q0q0 - q1q1 - q2q2 + q3q3 ;\n\n  ex = (ay*vz - az*vy) ;                           \t\t\t\t\t\n  ey = (az*vx - ax*vz) ;\n  ez = (ax*vy - ay*vx) ;\n\n  exInt = exInt + ex * Ki;\t\t\t\t\t\t\t\t \n  eyInt = eyInt + ey * Ki;\n  ezInt = ezInt + ez * Ki;\n\n  gx = gx + Kp*ex + exInt;\t\t\t\t\t   \t\t\t\t\t\t\t\n  gy = gy + Kp*ey + eyInt;\n  gz = gz + Kp*ez + ezInt;\t\t\t\t   \t\t\t\t\t\t\t\n\t\t\t\t\t   \n  q0 = q0 + (-q1*gx - q2*gy - q3*gz)*halfT;\n  q1 = q1 + (q0*gx + q2*gz - q3*gy)*halfT;\n  q2 = q2 + (q0*gy - q1*gz + q3*gx)*halfT;\n  q3 = q3 + (q0*gz + q1*gy - q2*gx)*halfT;\n\n  norm = sqrt(q0*q0 + q1*q1 + q2*q2 + q3*q3);\n  q0 = q0 / norm;\n  q1 = q1 / norm;\n  q2 = q2 / norm;\n  q3 = q3 / norm;\n\nPitch  = asin(-2 * q1 * q3 + 2 * q0* q2)* 57.3; // pitch\nRoll = atan2(2 * q2 * q3 + 2 * q0 * q1, -2 * q1 * q1 - 2 * q2* q2 + 1)* 57.3; // roll" "融合，四元数计算姿态"("q0"=w363, "q1"=w378, "q2"=w377, "q3"=w376, "exInt"=w375, "eyInt"=w374, "ezInt"=w373, "gx"=w350, "gy"=w361, "gz"=w360, "ax"=w351, "ay"=w356, "az"=w362, "Ki"=0.005 ("输入变量"), "Kp"=8.0 ("输入变量"), "halfT"=w354) -> ("q0"=w364:dbl, "q1"=w365:dbl, "q2"=w366:dbl, "q3"=w367:dbl, "exInt"=w368:dbl, "eyInt"=w369:dbl, "ezInt"=w370:dbl, "Pitch"=w352:dbl, "Roll"=w347:dbl)
          "roll" <- w347
          n129 = Bundle By Name(cluster=w372, "q0"=w364, "q1"=w365, "q2"=w366, "q3"=w367, "exInt"=w368, "eyInt"=w369, "ezInt"=w370) -> (w371:T9)
        }
      }
      n130 = feedback-in #9(w285) -> ()
      n131 = feedback #9(T9 {"q0"=1.0, "q1"=0.0, "q2"=0.0, "q3"=0.0, "exInt"=0.0, "eyInt"=0.0, "ezInt"=0.0}) -> (w286:T9)
      n132 = local read "Y axis"() -> (w221:i32)
      n133 = local read "X axis"() -> (w222:i32)
      n134 = To Single Precision Float(number=w221) -> (single precision float=w220:sgl)
      n135 = To Single Precision Float(number=w222) -> (single precision float=w223:sgl)
      n136 = Divide(x=w220, y=sgl 6000.0) -> (x/y=w218:sgl)
      n137 = Divide(x=w223, y=sgl -6000.0) -> (x/y=w219:sgl)
      n138 = To Single Precision Float(number=w254) -> (single precision float=w258:sgl)
      n139 = To Single Precision Float(number=w257) -> (single precision float=w279:sgl)
      n140 = Bundle By Name(cluster=w281, "Roll"=w258, "Pitch"=w279, "Yaw"=w249) -> (w265:cluster{"Roll":sgl, "Pitch":sgl, "Yaw":sgl})
      n141 = Bundle(w218, "Pitch"=w257) -> (→"Pitch: 控制\\反馈":cluster{sgl, "Pitch":dbl})  [unwired: 1 in]
      n142 = Bundle(w219, "Roll"=w254) -> (→"Roll: 控制\\反馈":cluster{sgl, "Roll":dbl})  [unwired: 1 in]
      n143 = Bundle By Name(cluster=w260, "Z"="滑动杆", "X"=w219, "Y"=w218) -> (w259:cluster{"X":sgl, "Y":sgl, "Z":sgl})
      n144 = Bundle("GYR_I_Z"=w249) -> (→"Yaw: 控制\\反馈":cluster{"GYR_I_Z":sgl})  [unwired: 1 in]
      n145 = Subtract(x=w259, y=w265) -> (x-y=w273:cluster{sgl, sgl, sgl})
      n146 = local read "油门"() -> (w232:u16)
      n147 = flat-sequence {
        tunnel: w273 -> [w344]
        tunnel: w247 -> [w343]
        tunnel: [w336] -> w264
        tunnel: [w335] -> w263
        tunnel: [w334] -> w261
        tunnel: w271 -> [w333]
        tunnel: [w329] -> w269
        tunnel: [w328] -> w268
        tunnel: [w327] -> w267
        tunnel: w265 -> [w326]
        tunnel: w232 -> [w322]
        tunnel: [w319] -> w262
        tunnel: [w305] -> w243
        tunnel: [w312] -> w238
        tunnel: [w311] -> w237
        tunnel: [w310] -> w236
        tunnel: "滑动杆" -> [w308]
        tunnel: w202 -> [w305]
        frame #0 {
          n148 = Unbundle By Name(w343) -> ("GX"=w342:sgl, "GY"=w341:sgl, "GZ"=w340:sgl)
          n149 = Unbundle(w344) -> (w338:sgl, w339:sgl, w337:sgl)
          n150 = Unbundle(w326) -> ("Roll"=w324:sgl, "Pitch"=w325:sgl, "Yaw"=w323:sgl)
          n151 = Unbundle By Name(w333) -> ("EI_Roll"=w332:sgl, "EI_Pitch"=w331:sgl, "EI_Yaw"=w330:sgl)
          n152 = Divide(x=500.0 ("输入变量"), y="I") -> (x/y=w318:dbl)
          n153 = formula code="float Roll, Pitch, Yaw, Yaw_PD_Part, Yaw_StickSet;\n\n\n\n//Roll方向PID\n//计算比例\nRoll = RP_P * ER;\n//计算积分\n//if(Q_Roll > -0.1 && Q_Roll < 0.1)\n//{\n //     EI_Roll = 0;\n//}\n//else\n//{\n       EI_Roll += ER;\n//}\nif(EI_Roll > RP_MAX)\n       EI_Roll = RP_MAX;\nif(EI_Roll < (0 - RP_MAX))\n       EI_Roll = - RP_MAX;\n//加上积分\nRoll += RP_I * EI_Roll;\n//加上微分\nRoll -= RP_D * GX;\n\n//Pitch方向PID\n//计算比例\nPitch = RP_P * EP;\n//计算积分\n//if(Q_Pitch > -0.1 && Q_Pitch < 0.1)\n//{\n //     EI_Pitch = 0;\n//}\n//else\n//{\n     EI_Pitch += EP;\n//}\nif(EI_Pitch > RP_MAX)\n       EI_Pitch = RP_MAX;\nif(EI_Pitch < (0 - RP_MAX))\n       EI_Pitch = - RP_MAX;\n//加上积分\nPitch += RP_I * EI_Pitch;\n//加上微分\nPitch -= RP_D * GY;\n\n//Yaw方向PID\nYaw_PD_Part = GZ * 2 * Yaw_P + Q_Yaw * Yaw_I / 2;\nif(Thr > 100){\nYaw_StickSet = StickYawP * (StickYaw * abs(StickYaw)) / 512 + StickYawP * StickYaw / 4;\n}\nYaw = Yaw_PD_Part - Yaw_StickSet * STICK_GAIN;\nif(Yaw > 1000) Yaw = 1000;\nif(Yaw < -1000) Yaw = -1000;\n\n//X型电机分配算法，与传感器及电机的安装位置相关\n//MP1 = Thr + Roll - Pitch - Yaw;\n//MP2 = Thr + Roll + Pitch + Yaw;\n//MP3 = Thr - Roll + Pitch - Yaw;\n//MP0 = Thr - Roll - Pitch + Yaw;\n\n//十型电机分配算法\nMP0 = Thr - Roll + Yaw;\nMP1 = Thr - Pitch - Yaw;\nMP2 = Thr + Roll + Yaw;\nMP3 = Thr + Pitch - Yaw;" ("公式节点")("GX"=w342, "GY"=w341, "GZ"=w340, "ER"=w338, "EP"=w339, "EY"=w337, "Thr"=w322, "EI_Roll"=w332, "EI_Pitch"=w331, "EI_Yaw"=w330, "RP_P"="P", "RP_I"="I", "RP_D"="D", "Q_Roll"=w324, "Q_Pitch"=w325, "Q_Yaw"=w323, "RP_MAX"=w318, "Yaw_P"="Yaw_D", "Yaw_I"="Yaw_P", "Yaw_D"="Yaw_I", "Yaw_MAX"=10.0 ("输入变量"), "StickYaw"=w308, "StickYawP"=0.0 ("输入变量"), "STICK_GAIN"=4.0 ("输入变量")) -> ("MP0"=w336:dbl, "MP1"=w335:dbl, "MP2"=w319:dbl, "MP3"=w334:dbl, "EI_Roll"=w329:sgl, "EI_Pitch"=w328:sgl, "EI_Yaw"=w327:sgl, "Roll"=w312:dbl, "Pitch"=w311:dbl, "Yaw"=w310:dbl)
        }
      }
      n154 = local read "摇杆按键"() -> (w235:bool[])
      n155 = Index Array(array=w235, index #1=6 ("索引"), index #2=7 ("索引"), index #3=2 ("索引"), index #4=1 ("索引")) -> (element #1=w216:bool, element #2=w215:bool, element #3=w207:bool, element #4=w206:bool)
      n156 = Compound Arithmetic op=OR(w216, w215) -> (w214:bool)
      n157 = Or(x="停止调试", y=w214) -> (x .or. y?=w234:bool)
      n158 = case shown="True" w207 {
        tunnel: w205 -> [_ w303]
        frame False {
        }
        frame True {
          n159 = call "MotorEnCtrl.vi"("MotorEN?(F)"=FALSE, "FPGA VI引用输入"=w303) -> ()  [unwired: 8 in, 2 out]
        }
      }
      n160 = feedback #10(w272) -> (w271:T8)
      n161 = case shown="True" w206 {
        tunnel: w205 -> [_ w300]
        frame False {
        }
        frame True {
          n162 = local read "油门"() -> (w299:u16)
          n163 = Less?(x=w299, y=u16 200) -> (x < y?=w298:bool)
          n164 = case shown="True" w298 {
            tunnel: w300 -> [_ w301]
            frame False {
            }
            frame True {
              n165 = call "MotorEnCtrl.vi"("MotorEN?(F)"=TRUE, "FPGA VI引用输入"=w301) -> ()  [unwired: 8 in, 2 out]
            }
          }
        }
      }
      n166 = To Unsigned Word Integer(number=w264) -> (unsigned 16bit integer=w197:u16)
      n167 = To Unsigned Word Integer(number=w263) -> (unsigned 16bit integer=w195:u16)
      n168 = To Unsigned Word Integer(number=w262) -> (unsigned 16bit integer=w193:u16)
      n169 = To Unsigned Word Integer(number=w261) -> (unsigned 16bit integer=w191:u16)
      n170 = Bundle By Name(cluster=T8 {"EI_Roll"=0.0, "EI_Pitch"=0.0, "EI_Yaw"=0.0} ("EI"), "EI_Roll"=w269, "EI_Pitch"=w268, "EI_Yaw"=w267) -> (w266:T8)
      n171 = feedback-in #10(w266) -> ()
      n172 = Multiply(x=w195, y=u16 2) -> (x*y=w194:u16)
      n173 = call "PWMFeedDog.vi"("ErrorIn(no error)"=w243, "FPGA VI引用输入"=w205) -> ("ErrorOut"=w278:errorcluster, "FPGA VI引用输出"=w276:refnum<k20>)  [unwired: 8 in]
      n174 = Multiply(x=w197, y=u16 2) -> (x*y=w196:u16)
      n175 = Multiply(x=w193, y=u16 2) -> (x*y=w192:u16)
      n176 = Multiply(x=w191, y=u16 2) -> (x*y=w190:u16)
      n177 = Bundle By Name(cluster=T1 {"PWM0"=0, "PWM1"=0, "PWM2"=0, "PWM3"=0} ("MotorPower"), "PWM0"=w196, "PWM1"=w194, "PWM2"=w192, "PWM3"=w190) -> (w274:T1)
      "输出簇" <- w274
      n178 = call "PutMotorPower.vi"("ErrorIn(no error)"=w278, "MotorPower"=w274, "FPGA VI引用输入"=w276) -> ("ErrorOut"=w277:errorcluster, "FPGA VI引用输出"=w209:refnum<k20>)  [unwired: 7 in]
      n179 = node-c288() -> ()  [unwired: 1 in, 1 out]
      "Roll计算后数值" <- w238
      "Pitch计算后数值" <- w237
      "Yaw计算后数值" <- w236
    }
    n180 = local read "停止调试"() -> (w46:bool)
    n181 = local read "摇杆按键"() -> (w50:bool[])
    n182 = Index Array(array=w50, index=7 ("索引")) -> (element=w48:bool)
    n183 = Or(x=w48, y=w46) -> (x .or. y?=w47:bool)
    n184 = node-c288(w62) -> ()  [unwired: 1 out]
  }
  n185 = Obtain Notifier "获取通知器引用"(notification data type="" ("data out"), error in (no error)=w6) -> (notifier out=w7:refnum<notifier>, error out=w12:errorcluster)  [unwired: 2 in, 1 out]
  n186 = UDP Open "打开UDP"(8:w12, 11:u16 61557 ("port")) -> (port=w13:refnum<k16>, 0:w11:errorcluster)  [unwired: 3 in, 1 out]
  n187 = while {
    tunnel: w7 -> [w480]
    stop <- w478 stop-if-true
    w464 = 0
    w456 = i16 0
    n188 = Wait on Notification "等待通知"(notifier=w480) -> (notification=w479:string)  [unwired: 3 in, 3 out]
    n189 = String To Byte Array(string=w479) -> (unsigned byte array=w432:u8[])
    "Buffer In" <- w432
    n190 = Index Array(array=w432) -> (element #3=w440:u8, element #4=w441:u8, element #5=w442:u8, element #6=w443:u8, element #7=w444:u8, element #8=w445:u8, element #9=w446:u8, element #10=w447:u8, element #11=w448:u8, element #12=w449:u8, element #13=w460:u8, element #14=w461:u8, element #15=→"小方向":u8, element #16=w450:u8, element #17=w451:u8, element #18=w453:u8, element #19=w452:u8)  [unwired: 19 in, 2 out]
    n191 = Join Numbers(hi=w450, lo=w451) -> ((hi.lo)=w454:u16)
    n192 = Join Numbers(hi=w453, lo=w452) -> ((hi.lo)=w455:u16)
    n193 = Join Numbers(hi=w440, lo=w441) -> ((hi.lo)=→"油门":u16)
    n194 = Join Numbers(hi=w442, lo=w443) -> ((hi.lo)=w435:u16)
    n195 = Join Numbers(hi=w444, lo=w445) -> ((hi.lo)=w434:u16)
    n196 = Join Numbers(hi=w446, lo=w447) -> ((hi.lo)=w437:u16)
    n197 = Join Numbers(hi=w448, lo=w449) -> ((hi.lo)=w438:u16)
    n198 = Join Numbers(hi=w460, lo=w461) -> ((hi.lo)=w462:u16)
    n199 = Type Cast(type=w456, x=w454) -> (*(type *) &x=w457:i16)
    n200 = Type Cast(type=w456, x=w455) -> (*(type *) &x=w458:i16)
    n201 = Join Numbers(hi=w435, lo=w434) -> ((hi.lo)=w436:u32)
    n202 = Join Numbers(hi=w437, lo=w438) -> ((hi.lo)=w439:u32)
    n203 = To Single Precision Float(number=w457) -> (single precision float=w467:sgl)
    n204 = To Single Precision Float(number=w458) -> (single precision float=w468:sgl)
    n205 = Number To Boolean Array(number=w462) -> (Boolean array=→"摇杆按键":bool[])
    n206 = Type Cast(type=w464, x=w436) -> (*(type *) &x=w476:i32)
    "X axis" <- w476
    n207 = Type Cast(type=w464, x=w439) -> (*(type *) &x=w477:i32)
    "Y axis" <- w477
    n208 = Multiply(x=w467, y=sgl 0.1) -> (x*y=w470:sgl)
    n209 = Multiply(x=w468, y=sgl 0.1) -> (x*y=w469:sgl)
    n210 = Bundle By Name(cluster=T2 {"ACC_OFFSET_X"=0.0, "ACC_OFFSET_Y"=0.0, "ACC_OFFSET_Z"=0.0} ("ACCADJ"), "ACC_OFFSET_X"=w470, "ACC_OFFSET_Y"=w469) -> (w466:T2)
    n211 = Build Array(w476) -> (w474:i32[])
    n212 = Build Array(w477) -> (w475:i32[])
    n213 = Bundle(w474, w475) -> (→"XY图":cluster{i32[], i32[]})  [unwired: 1 in]
    n214 = local read "停止调试"() -> (w478:bool)
    n215 = local write "ACCADJ"(w466) -> ()
  }
  n216 = while {
    tunnel: w7 -> [w488]
    tunnel: w13 -> [w486]
    tunnel: w11 -> [w485]
    tunnel: [w484] -> w10
    tunnel: [w483] -> w9
    tunnel: [w482] -> w8
    stop <- w481 stop-if-true
    n217 = UDP Read "读取UDP数据"(connection ID=w486, 8:w485) -> (data out=w487:string, error out=w482:errorcluster, 3:w483:refnum<k16>)  [unwired: 2 in, 2 out]
    n218 = Send Notification "发送通知"(notification=w487, notifier=w488) -> (notifier out=w484:refnum<notifier>)  [unwired: 1 in, 1 out]
    n219 = local read "停止调试"() -> (w481:bool)
  }
  n220 = Release Notifier "释放通知器引用"(notifier=w10) -> ()  [unwired: 2 in, 3 out]
  n221 = UDP Close "关闭UDP"(connection ID=w9, 8:w8) -> ()  [unwired: 2 out]
  n222 = call "MotorEnCtrl.vi"("ErrorIn(no error)"=w28, "MotorEN?(F)"=FALSE, "FPGA VI引用输入"=w29) -> ("ErrorOut"=w26:errorcluster, "FPGA VI引用输出"=w27:refnum<k20>)  [unwired: 7 in]
  n223 = flat-sequence {
    tunnel: w26 -> [w490]
    tunnel: [w490] -> w33
    frame #0 {
      n224 = Wait (ms)(milliseconds to wait=u32 200 ("等待时间（毫秒）")) -> ()  [unwired: 1 out]
    }
  }
  n225 = call "PWMOutputEnControl.vi"("ErrorIn(no error)"=w33, "OutEN?(F)"=FALSE, "FPGA VI引用输入"=w27) -> ("ErrorOut"=w35:errorcluster, "FPGA VI引用输出"=w36:refnum<k20>)  [unwired: 7 in]
  n226 = call "MPUAtutoReadOff.vi"("ErrorIn(no error)"=w35, "FPGA VI引用输入"=w36) -> ("ErrorOut"=w37:errorcluster, "FPGA VI引用输出"=w38:refnum<k20>)  [unwired: 8 in]
  n227 = xnode "关闭FPGA VI引用"("FPGA VI引用输入"=w38, "错误输入"=w37) -> ()  [unwired: 1 out]
